vi "FITS hdr pad length.vi"(8 "error in (no error)":errorcluster, 11 "Header":string) -> (0 "error out":errorcluster, 3 "Padded Header":string)   [LabVIEW 2020]
panel:
  out "x/y":dbl
  out "length":i32
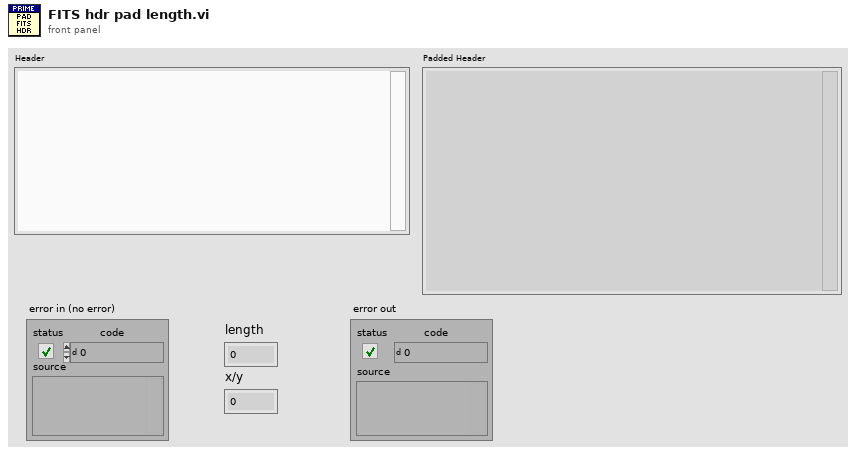
[diagram p1: front panel]
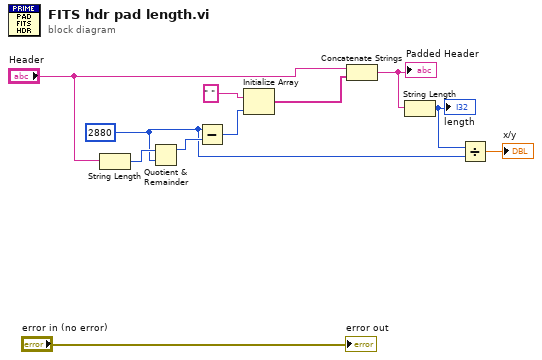
[diagram p0: block diagram]
diagram:
  w2 = 2880
  n1 = String Length(string="Header") -> (length=w10:i32)
  n2 = Quotient & Remainder(x=w10, y=w2) -> (x-y*floor(x/y)=w5:i32)  [unwired: 1 out]
  n3 = Subtract(x=w2, y=w5) -> (x-y=w4:i32)
  n4 = Initialize Array(" ", w4) -> (w7:string[])
  n5 = Concatenate Strings("Header", w7) -> (w6:string)
  "Padded Header" <- w6
  n6 = String Length(string=w6) -> (length=w3:i32)
  "length" <- w3
  n7 = Divide(x=w3, y=w2) -> (x/y=→"x/y":dbl)
  "error out" <- "error in (no error)"
